vi "TPI freq rounder.vi"(1 "input time (s)":dbl) -> (0 "rounded time (s)":dbl)   [LabVIEW 2017]
panel:
  out "int numCycles":i32
  out "numCycles":dbl
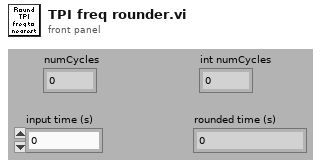
[diagram p1: front panel]
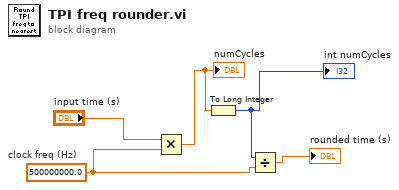
[diagram p0: block diagram]
diagram:
  w1 = 500000000.0  # clock freq (Hz)
  n1 = Multiply(x="input time (s)", y=w1) -> (x*y=w4:dbl)
  "numCycles" <- w4
  n2 = To Long Integer(number=w4) -> (32bit integer=w2:i32)
  "int numCycles" <- w2
  n3 = Divide(x=w2, y=w1) -> (x/y=→"rounded time (s)":dbl)
